vi "LVH5Rclose.vi"   [LabVIEW 2017]
doc: "Closes an HDF5 Reference object"
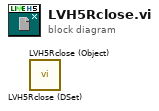
[diagram p0: block diagram]
diagram:
  n1 = call <vilib>:"LVH5Rclose (DSet).vi"() -> ()  [unwired: 9 in, 1 out]
  n2 = call <vilib>:"LVH5Rclose (Object).vi"() -> ()  [unwired: 9 in, 1 out]
